vi "String Indicator.vi"(10 "String Indicator":string) -> (3 "String Indicator Event out":refnum<class "String Indicator Event.lvclass">)   [LabVIEW 2021, in "String Indicator Event.lvlib" / "String Indicator Event.lvclass"]
uses:
  String Indicator Event.lvclass
  String Indicator Event.lvclass/String Indicator Event.ctl
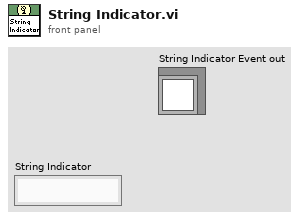
[diagram p1: front panel]
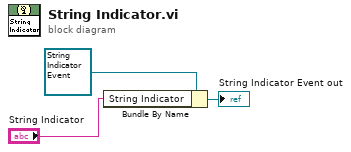
[diagram p0: block diagram]
diagram:
  n1 = Bundle By Name(cluster=refnum<class "String Indicator Event.lvclass"> refnum ("String Indicator Ref.lvlib:String Indicator Msg.lvclass"), "String Indicator"="String Indicator") -> (→"String Indicator Event out":refnum<class "String Indicator Event.lvclass">)
